vi "Create VI function name.vi"(8 "error in (no error)":errorcluster, 11 "y":string) -> (0 "error out":errorcluster, 3 "String":string)   [LabVIEW 2025, in "Scripting Server.lvlib" / "Tools.lvlib"]
uses:
  Tools.lvlib
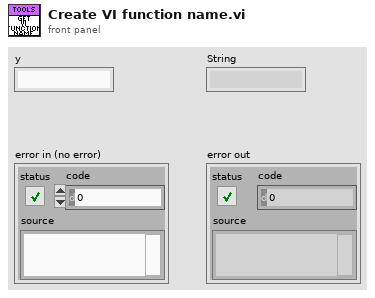
[diagram p1: front panel]
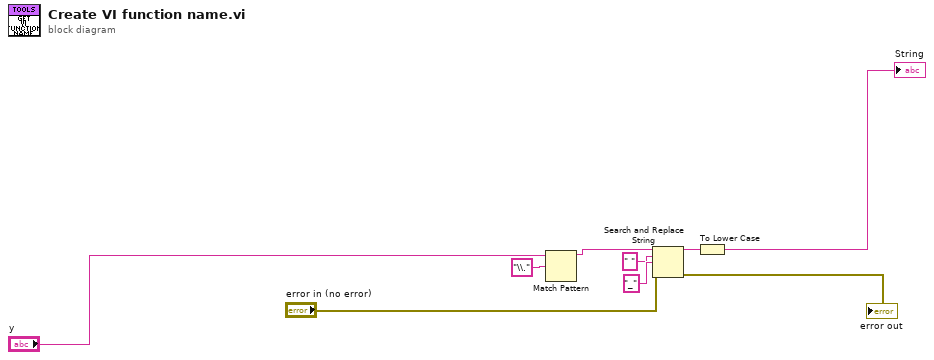
[diagram p0: block diagram]
diagram:
  n1 = Match Pattern(string="y", regular expression="\\." ("string")) -> (before substring=w1:string)  [unwired: 1 in, 3 out]
  n2 = Search and Replace String(input string=w1, search string=" ", replace string="_" ("replace string (\"\")"), error in="error in (no error)") -> (result string=w6:string, error out=→"error out":errorcluster)  [unwired: 4 in, 2 out]
  n3 = To Lower Case(string=w6) -> (all lower case string=→"String":string)
